vi "Control Start Recording.vi"   [LabVIEW 2020]
uses:
  Framework/Robot Global Data.vi
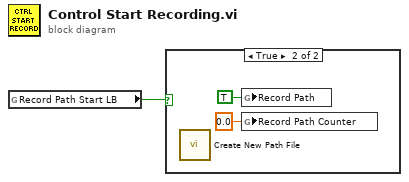
[diagram p0: block diagram]
diagram:
  n1 = global read "Robot Global Data.vi" "Record Path Start LB"() -> (w1:bool)
  n2 = case shown="True" w1 {
    frame False {
    }
    frame True {
      n3 = call "Create New Path File.vi"() -> ()  [unwired: 12 in]
      n4 = global write "Robot Global Data.vi" "Record Path"(TRUE ("Record Path")) -> ()
      n5 = global write "Robot Global Data.vi" "Record Path Counter"(0.0 ("Record Path Counter")) -> ()
    }
  }
